vi "ETH_11.vi"(7 "Enum":enum16{"Read", "Write"}(ring), 8 "error in":errorcluster, 11 "ETH 11":T1) -> (0 "error out":errorcluster, 3 "ETH_11":T1)   [LabVIEW 2022 SP3]
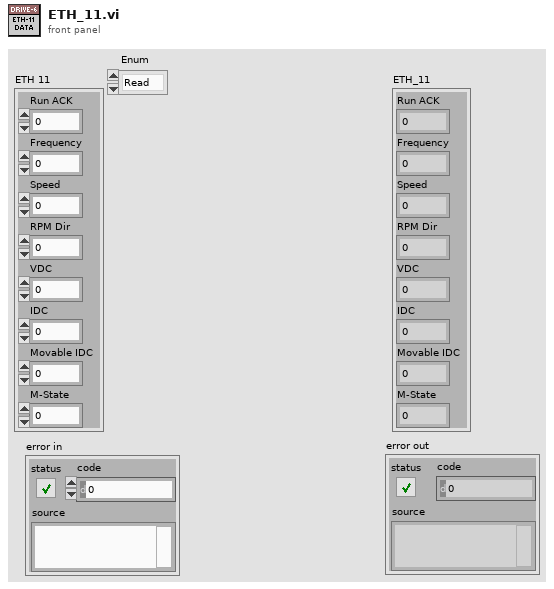
[diagram p1: front panel]
types:
  T1 = cluster{"Run ACK":dbl, "Frequency":dbl, "Speed":dbl, "RPM Dir":dbl, "VDC":dbl, "IDC":dbl, "Movable IDC":dbl, "M-State":dbl}
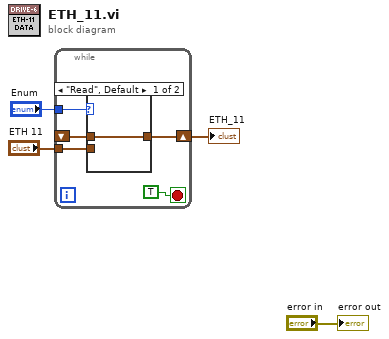
[diagram p0: block diagram]
diagram:
  n1 = while {
    tunnel: "Enum" -> [w9]
    tunnel: "ETH 11" -> [w7]
    shift-right: [w6] -> w1
    shift-left: _ -> [w5]
    stop <- TRUE stop-if-true
    n2 = case shown="\"Read\", Default" w9 {
      tunnel: w7 -> [_ w11]
      tunnel: [w10 w11] -> w6
      tunnel: w5 -> [w10 _]
      frame "Read", Default {
      }
      frame "Write" {
      }
    }
  }
  "ETH_11" <- w1
  "error out" <- "error in"
